vi "parse_InertiaStamped_roslv.vi"(4 "error in":errorcluster, 7 "msg in":string) -> (0 "error out":errorcluster, 1 "Inertia":T1, 2 "Header":T2, 3 "msg out":string)   [LabVIEW 2014]
doc: "Parses a message into an inertia stamped"
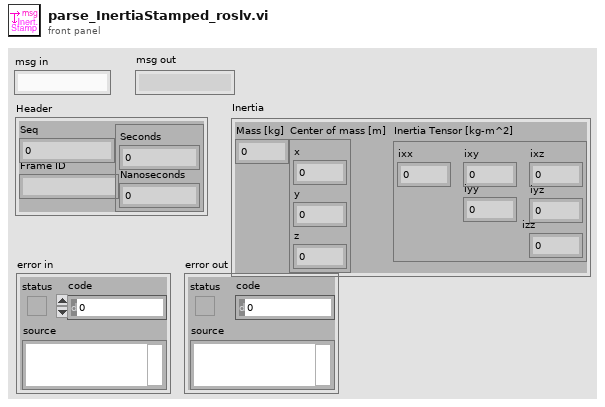
[diagram p1: front panel]
types:
  T1 = cluster{"Mass [kg]":dbl, "Center of mass [m]":cluster{"x":dbl, "y":dbl, "z":dbl}, "Inertia Tensor [kg-m^2]":cluster{"ixx":dbl, "ixy":dbl, "ixz":dbl, "iyy":dbl, "iyz":dbl, "izz":dbl}}
  T2 = cluster{"Seq":u32, "Frame ID":string, "Timestamp":cluster{"Seconds":i32, "Nanoseconds":i32}}
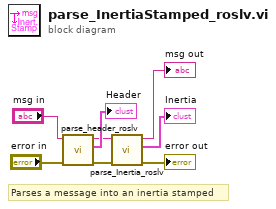
[diagram p0: block diagram]
diagram:
  # "Parses a message into an inertia stamped"
  n1 = call "parse_header_roslv.vi"("error in"="error in", "msg in"="msg in") -> ("error out"=w3:errorcluster, "Header"=→"Header":T2, "msg out"=w4:string)  [unwired: 3 in]
  n2 = call "parse_Inertia_roslv.vi"("error in"=w3, "msg in"=w4) -> ("error out"=→"error out":errorcluster, "Inertia"=→"Inertia":T1, "msg out"=→"msg out":string)  [unwired: 3 in]
